vi "Initialize.vi"(0 "VISA resource name":refnum<visa-resource-name>, 5 "Serial Configuration":T1={"Baud Rate"=38400, "Parity"=0, "Data Bits"=8, "Stop Bits"=10, "Flow Control"=0} {"Flow Control" items=["None", "XON/XOFF", "RTS/CTS", "XON/XOFF & RTS/CTS", "DTR/DSR", "XON/XOFF & DTR/DSR"]; "Stop Bits" items=["1.0"=10, "1.5"=15, "2.0"=20]; "Data Bits" items=["7"=7, "8"=8]; "Parity" items=["None", "Odd", "Even", "Mark", "Space"]; "Baud Rate" items=["300"=300, "600"=600, "1200"=1200, "2400"=2400, "4800"=4800, "9600"=9600, "19200"=19200, "38400"=38400]}, 9 "Reset (True)":bool=TRUE, 11 "error in (no error)":errorcluster, 12 "Timeout (10000 ms)":u32=10000) -> (4 "VISA resource name out":refnum<visa-resource-name>, 6 "Firmware Version":string, 15 "error out":errorcluster)   [LabVIEW 2020, in "eec EST 300.lvlib"]
doc: "Establishes communication with the instrument and optionally performs an instrument identification query and/or an instrument reset. It also places the instrument in a default state needed for other instrument driver operations. Call this VI before other instrument driver VIs for this instrument. Generally, you need to call the Initialize VI only once at the beginning of an application."
uses:
  <instrlib>/eec EST 300/eec EST 300.lvlib
  <instrlib>/eec EST 300/Private/Extended User Data.ctl
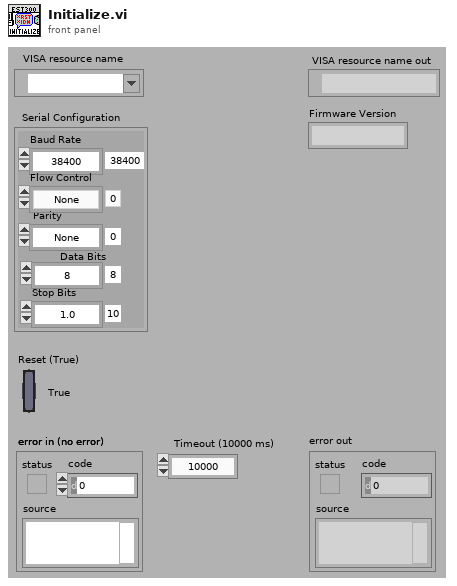
[diagram p1: front panel]
types:
  T1 = cluster{"Baud Rate":u32, "Parity":u16, "Data Bits":u16, "Stop Bits":u16, "Flow Control":u16}
  T2 = typedef "eec EST 300.lvlib/Extended User Data.ctl" = cluster{"Firmware Version":string, "Instrument Model":string}
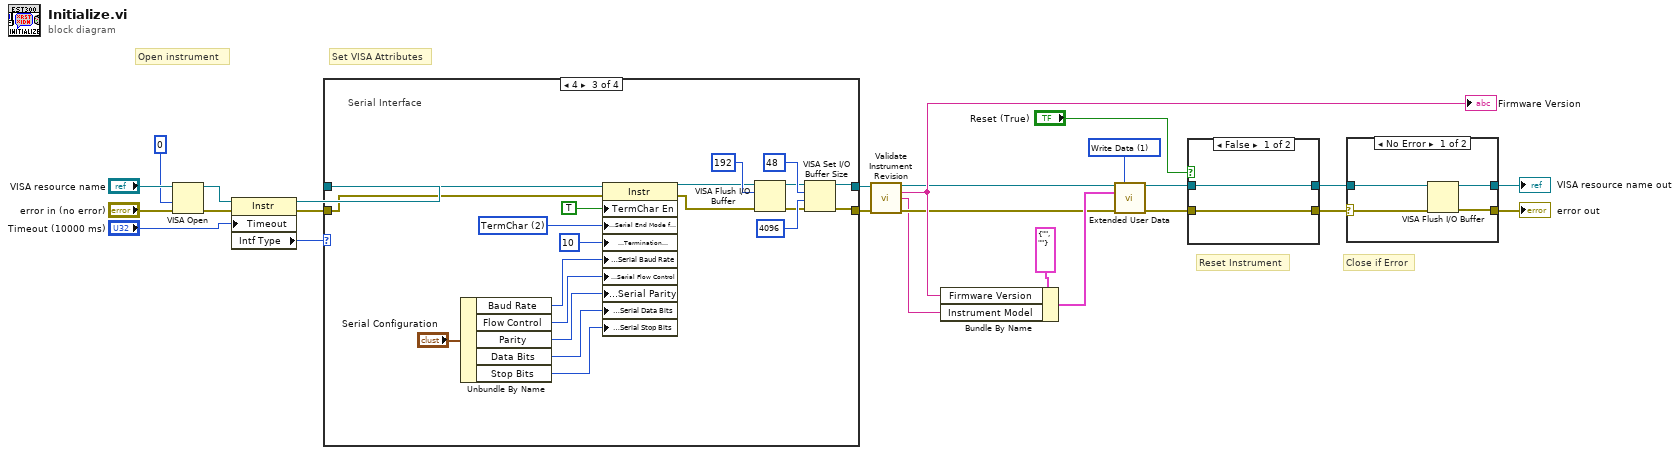
[diagram p0: block diagram]
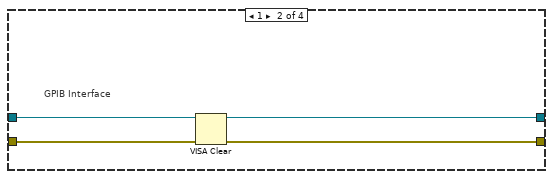
[diagram p3: hidden frame]
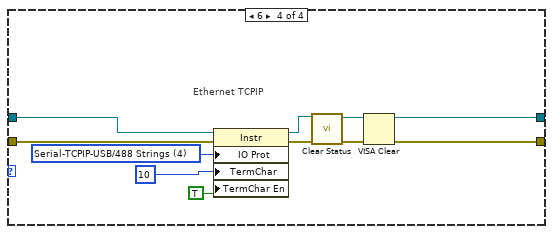
[diagram p4: hidden frame]
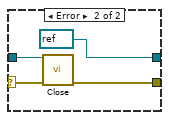
[diagram p5: hidden frame]
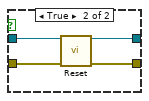
[diagram p6: hidden frame]
diagram:
  w11 = u16 1 items=["Read Data", "Write Data", "Clear Data", "Clear ALL Data"] ("Action")
  # "Set VISA Attributes"
  # "Close if Error"
  # "Reset Instrument"
  # "Open instrument"
  n1 = VISA Open(access mode=u32 0, error in (no error)="error in (no error)", VISA resource name="VISA resource name") -> (VISA resource name=w22:refnum<visa-resource-name>, error out=w21:errorcluster)  [unwired: 2 in]
  n2 = property on="Property Node" class="Instr"(reference=w22, error in=w21, "Timeout"="Timeout (10000 ms)") -> (reference out=w16:refnum<visa-resource-name>, error out=w15:errorcluster, "Intf Type"=w14:u16)
  n3 = case shown="4" w14 {
    tunnel: [w27 w29 w36 w57] -> w3
    tunnel: [w26 w28 w35 w56] -> w2
    tunnel: w16 -> [w27 w30 w46 w62]
    tunnel: w15 -> [w26 w31 w45 w59]
    frame Default {
    }
    frame 1 {
      # "GPIB Interface"
      n4 = VISA Clear(VISA resource name=w30, error in (no error)=w31) -> (VISA resource name out=w29:refnum<visa-resource-name>, error out=w28:errorcluster)
    }
    frame 4 {
      w42 = u16 2 items=["None", "Last Bit", "TermChar"] ("Serial Settings:End Mode for Reads")
      # "Serial Interface"
      n5 = Unbundle By Name("Serial Configuration") -> ("Baud Rate"=w51:u32, "Flow Control"=w48:u16, "Parity"=w49:u16, "Data Bits"=w50:u16, "Stop Bits"=w47:u16)
      n6 = property class="Instr"(reference=w46, error in=w45, "TermChar En"=TRUE ("Enable Termination\nChar (T)"), "Serial Settings:Serial End Mode for Reads"=w42, "Message Based Settings:Termination Character"=u8 10 ("termination char\n(0xA = '\\n' = LF)"), "Serial Settings:Serial Baud Rate"=w51, "Serial Settings:Serial Flow Control"=w48, "Serial Settings:Serial Parity"=w49, "Serial Settings:Serial Data Bits"=w50, "Serial Settings:Serial Stop Bits"=w47) -> (reference out=w34:refnum<visa-resource-name>, error out=w33:errorcluster)
      n7 = VISA Flush I/O Buffer(VISA resource name=w34, mask (16)=u16 192, error in (no error)=w33) -> (VISA resource name out=w37:refnum<visa-resource-name>, error out=w38:errorcluster)
      n8 = VISA Set I/O Buffer Size(VISA resource name=w37, mask (16)=u16 48, size (4096)=u32 4096 ("size (0)"), error in (no error)=w38) -> (VISA resource name out=w36:refnum<visa-resource-name>, error out=w35:errorcluster)
    }
    frame 6 {
      w61 = u16 4 items=["Normal"=1, "VXI/FDC"=2, "GPIB/HS488"=3, "Serial-TCPIP-USB/488 Strings"=4, "USBTMC/Vendor-Specific"=5] ("Message Based Settings:IO Protocol")
      # "Ethernet TCPIP"
      n9 = property on="Property Node" class="Instr"(reference=w62, error in=w59, "IO Prot"=w61, "TermChar"=u8 10 ("Message Based Settings:Termination Character"), "TermChar En"=TRUE ("Message Based Settings:Termination Character Enable")) -> (reference out=w58:refnum<visa-resource-name>, error out=w54:errorcluster)
      n10 = call <instrlib>:"Clear Status.vi"("VISA resource name"=w58, "error in (no error)"=w54) -> ("VISA resource name out"=w55:refnum<visa-resource-name>, "error out"=w53:errorcluster)  [unwired: 12 in]
      n11 = VISA Clear(VISA resource name=w55, error in (no error)=w53) -> (VISA resource name out=w57:refnum<visa-resource-name>, error out=w56:errorcluster)
    }
  }
  n12 = call <instrlib>:"Validate Instrument Revision.vi"("VISA resource name"=w3, "error in (no error)"=w2) -> ("VISA resource name out"=w7:refnum<visa-resource-name>, "Firmware Version"=w9:string, "Instrument Model"=w1:string, "error out"=w5:errorcluster)  [unwired: 10 in]
  "Firmware Version" <- w9
  n13 = Bundle By Name(cluster=T2 {"Firmware Version"="", "Instrument Model"=""} ("User Data In"), "Firmware Version"=w9, "Instrument Model"=w1) -> (w8:T2)
  n14 = call <instrlib>:"Extended User Data.vi"("VISA resource name"=w7, "Action"=w11, "User Data In"=w8, "Error In (no error)"=w5) -> ("VISA resource name out"=w6:refnum<visa-resource-name>, "Error Out"=w4:errorcluster)  [unwired: 9 in, 1 out]
  n15 = case shown="False" "Reset (True)" {
    tunnel: w4 -> [w63 w65]
    tunnel: [w63 w67] -> w13
    tunnel: w6 -> [w64 w66]
    tunnel: [w64 w68] -> w18
    frame False {
    }
    frame True {
      n16 = call <instrlib>:"Reset.vi"("VISA resource name"=w66, "error in (no error)"=w65) -> ("VISA resource name out"=w68:refnum<visa-resource-name>, "error out"=w67:errorcluster)  [unwired: 12 in]
    }
  }
  n17 = case shown="No Error" w13 {
    selector: w13 -> [w70 w74]
    tunnel: w18 -> [w72 w75]
    tunnel: [w71 refnum<visa-resource-name> refnum ("VISA resource name out")] -> w20
    tunnel: [w69 w76] -> w19
    frame No Error {
      n18 = VISA Flush I/O Buffer(VISA resource name=w72, error in (no error)=w70) -> (VISA resource name out=w71:refnum<visa-resource-name>, error out=w69:errorcluster)  [unwired: 1 in]
    }
    frame Error {
      n19 = call <instrlib>:"Close.vi"("VISA resource name"=w75, "error in (no error)"=w74) -> ("error out"=w76:errorcluster)  [unwired: 13 in]
    }
  }
  "VISA resource name out" <- w20
  "error out" <- w19
